vi "get_content_at.vi"(5 "ignore IDs":bool, 6 "ID chain":string[](array[string]), 7 "attribute name":string, 8 "error in (no error)":errorcluster, 10 "key chain":string[](array[string]), 11 "Element in":refnum<class "XMLElement.lvclass">) -> (0 "error out":errorcluster, 1 "found?":bool, 2 "string":string, 3 "Element out":refnum<class "XMLElement.lvclass">)   [LabVIEW 2010, in "XMLElement.lvclass"]
uses:
  XMLElement.lvclass
  XMLElement.lvclass/XMLElement.ctl
  Program Files/National Instruments/LabVIEW 2010/resource/objmgr/DOMUserDefRef.rc
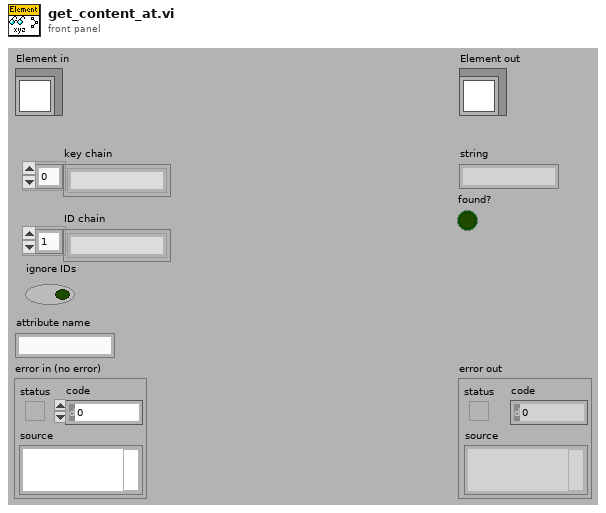
[diagram p1: front panel]
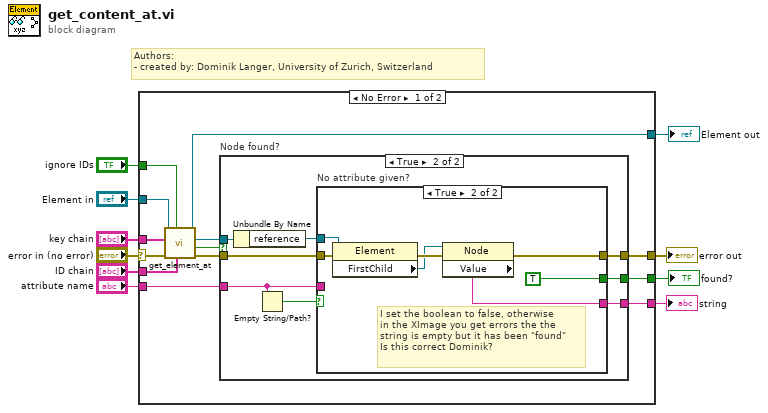
[diagram p0: block diagram]
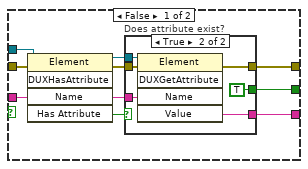
[diagram p3: hidden frame]
diagram:
  # "Authors: \n- created by: Dominik Langer, University of Zurich, Switzerland"
  n1 = case shown="No Error" "error in (no error)" {
    selector: "error in (no error)" -> [w20 w58]
    tunnel: [w23 w58] -> w9
    tunnel: [w18 w57] -> w7
    tunnel: "Element in" -> [w19 w57]
    tunnel: "key chain" -> [w11 _]
    tunnel: "ID chain" -> [w14 _]
    tunnel: "ignore IDs" -> [w13 _]
    tunnel: "attribute name" -> [w22 _]
    tunnel: [w21 _] -> w2
    tunnel: [w12 _] -> w1
    frame No Error {
      n2 = call "get_element_at.vi"("id chain"=w14, "ignore IDs"=w13, "error in (no error)"=w20, "key chain"=w11, "Element in"=w19) -> ("error out"=w16:errorcluster, "found?"=w15:bool, "element"=w17:refnum<class "XMLElement.lvclass">, "Element out"=w18:refnum<class "XMLElement.lvclass">)  [unwired: 3 in]
      n3 = case "Node found?" shown="True" w15 {
        selector: w15 -> [w24 _]
        tunnel: [w25 w33] -> w23
        tunnel: w22 -> [_ w28]
        tunnel: [_ w32] -> w21
        tunnel: w17 -> [_ w31]
        tunnel: w16 -> [w25 w29]
        tunnel: [w24 w26] -> w12
        frame False {
        }
        frame True {
          n4 = Unbundle By Name(w31) -> ("reference"=w30:refnum<k20>)
          n5 = Empty String/Path?(string/path=w28) -> (empty?=w27:bool)
          n6 = case "No attribute given?" shown="True" w27 {
            tunnel: [w42 w51] -> w33
            tunnel: w28 -> [w36 _]
            tunnel: [w41 w52] -> w32
            tunnel: w30 -> [w38 w56]
            tunnel: w29 -> [w40 w55]
            tunnel: [w34 TRUE] -> w26
            frame False {
              n7 = invoke class="Element" method="DUXHasAttribute"(reference=w38, error in=w40, "Name"=w36) -> (reference out=w37:refnum<k20>, error out=w39:errorcluster, "Has Attribute"=w35:bool)  [unwired: 2 in, 2 out]
              n8 = case "Does attribute exist?" shown="True" w35 {
                tunnel: [w43 w49] -> w42
                tunnel: [_ w48] -> w41
                tunnel: w39 -> [w43 w47]
                tunnel: w37 -> [_ w46]
                tunnel: w36 -> [_ w45]
                tunnel: [_ TRUE] -> w34
                frame False {
                }
                frame True {
                  n9 = invoke class="Element" method="DUXGetAttribute"(reference=w46, error in=w47, "Name"=w45) -> (error out=w49:errorcluster, "Value"=w48:string)  [unwired: 2 in, 3 out]
                }
              }
            }
            frame True {
              # "I set the boolean to false, otherwise\nin the XImage you get errors the the\nstring is empty but it has been \"found\"\nIs this correct Dominik?"
              n10 = property class="Element"(reference=w56, error in=w55) -> (error out=w54:errorcluster, "FirstChild"=w53:refnum<k20>)  [unwired: 1 out]
              n11 = property class="Node"(reference=w53, error in=w54) -> (error out=w51:errorcluster, "Value"=w52:string)  [unwired: 1 out]
            }
          }
        }
      }
    }
    frame Error {
    }
  }
  "error out" <- w9
  "Element out" <- w7
  "string" <- w2
  "found?" <- w1
